vi "Int 1D From Items.vi"(10 "Child Text":string[](array[string])) -> (2 "Number":i32[](array[numeric]))   [LabVIEW 2024]
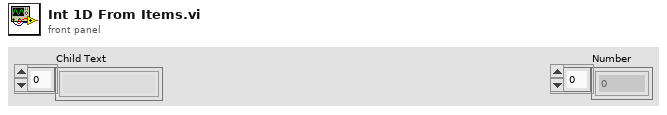
[diagram p1: front panel]
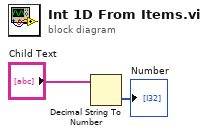
[diagram p0: block diagram]
diagram:
  n1 = Decimal String To Number(string="Child Text") -> (number=→"Number":i32[])  [unwired: 2 in, 1 out]
